vi "Check syntax.vi"(8 "error in":errorcluster, 11 "<single path ele>":string) -> (0 "error out":errorcluster)   [LabVIEW 2015]
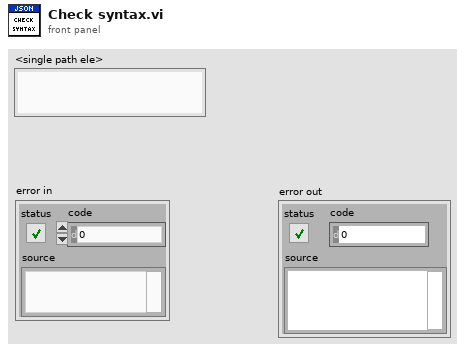
[diagram p1: front panel]
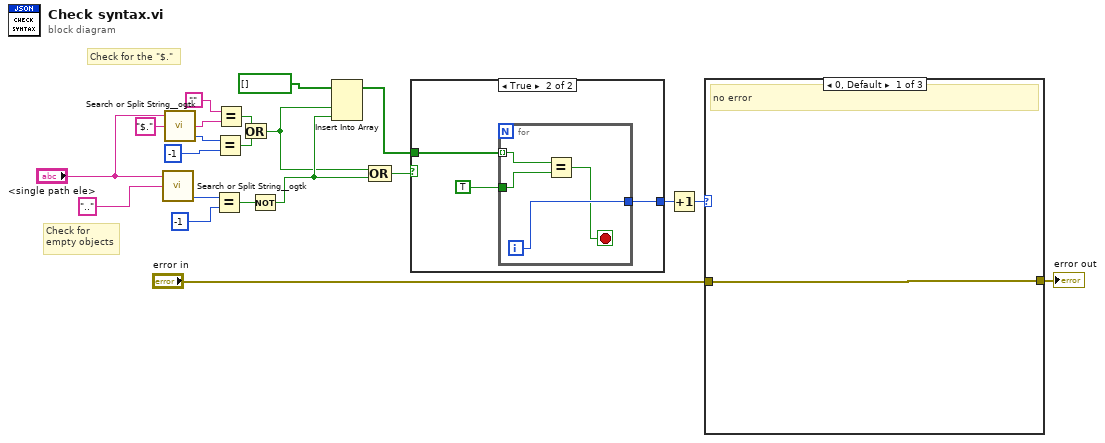
[diagram p0: block diagram]
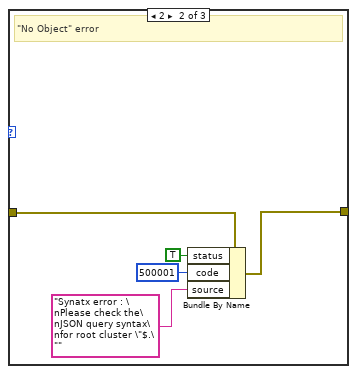
[diagram p2: hidden frame]
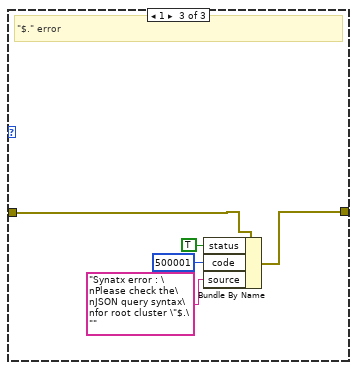
[diagram p3: hidden frame]
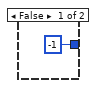
[diagram p4: hidden frame]
diagram:
  # "Check for\nempty objects"
  # "Check for the \"$.\""
  n1 = call <userlib>:"Search or Split String__ogtk.vi"("search string/char (-)"="..", "string"="<single path ele>") -> ("offset after match"=w20:i32)  [unwired: 1 in, 2 out]
  n2 = call <userlib>:"Search or Split String__ogtk.vi"("search string/char (-)"="$.", "string"="<single path ele>") -> ("offset after match"=w6:i32, "substring after match"=w2:string)  [unwired: 1 in, 1 out]
  n3 = Equal?(x=w20, y=-1) -> (x = y?=w18:bool)
  n4 = Equal?(x=w6, y=-1) -> (x = y?=w5:bool)
  n5 = Equal?(x="", y=w2) -> (x = y?=w4:bool)
  n6 = Or(x=w4, y=w5) -> (x .or. y?=w3:bool)
  n7 = Not(x=w18) -> (.not. x?=w12:bool)
  n8 = Insert Into Array(array=bool[] [], new element #1=w3, new element #2=w12) -> (w11:bool[])  [unwired: 1 in]
  n9 = Compound Arithmetic op=OR(w3, w12) -> (w14:bool)
  n10 = case shown="True" w14 {
    tunnel: w11 -> [_ w25]
    tunnel: [-1 w23] -> w10
    frame False {
    }
    frame True {
      n11 = for {
        tunnel: w25 -> [w28] mode=indexing
        tunnel: TRUE -> [w29]
        tunnel: [w27] -> w23
        i -> [w27]
        stop <- w26 stop-if-true
        n12 = Equal?(x=w28, y=w29) -> (x = y?=w26:bool)
      }
    }
  }
  n13 = Increment(x=w10) -> (x+1=w8:i32)
  n14 = case shown="0, Default" w8 {
    tunnel: "error in" -> [w30 w35 w40]
    tunnel: [w30 w31 w36] -> w7
    frame 0, Default {
      # "no error"
    }
    frame 2 {
      # "\"No Object\" error"
      n15 = Bundle By Name(cluster=w35, "status"=TRUE, "code"=500001, "source"="Synatx error : \nPlease check the\nJSON query syntax\nfor root cluster \"$.\"") -> (w31:errorcluster)
    }
    frame 1 {
      # "\"$.\" error"
      n16 = Bundle By Name(cluster=w40, "status"=TRUE, "code"=500001, "source"="Synatx error : \nPlease check the\nJSON query syntax\nfor root cluster \"$.\"") -> (w36:errorcluster)
    }
  }
  "error out" <- w7
